vi "Decode Error.vi"(9 "cancel byte":u8, 10 "status byte":u8) -> (0 "Status":T1, 1 "Error message":string, 2 "Bad status byte?":bool, 3 "Error occured?":bool)   [LabVIEW 2023, in "Digikrom DK24x.lvlib"]
doc: "Decodes the status byte returned by the instrument."
uses:
  Digikrom DK24x.lvlib
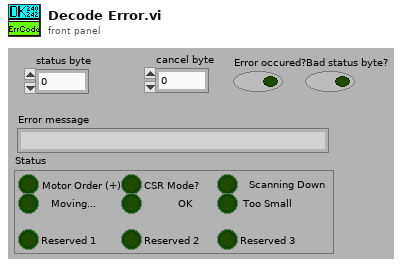
[diagram p1: front panel]
types:
  T1 = cluster{"Motor Order?":bool, "Reserved 1":bool, "CSR Mode?":bool, "Reserved 2":bool, "Scanning Up?":bool, "Too Large?":bool, "Already There?":bool, "Invalid Value?":bool, "Reserved 3":bool}
  T2 = cluster{"Boolean array[0]":bool, "Boolean array[1]":bool, "Boolean array[2]":bool, "Boolean array[3]":bool, "Boolean array[4]":bool, "Boolean array[5]":bool, "Boolean array[6]":bool, "Boolean array[7]":bool, "Boolean array[8]":bool}
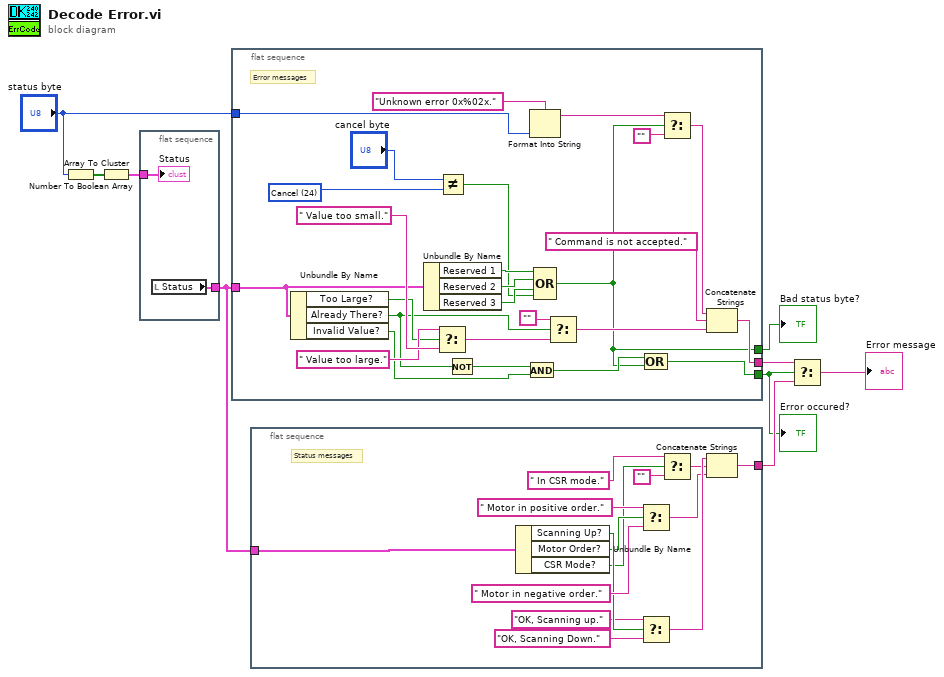
[diagram p0: block diagram]
diagram:
  n1 = Number To Boolean Array(number="status byte") -> (Boolean array=w7:bool[])
  n2 = Array To Cluster(array=w7) -> (cluster=w8:T2)
  n3 = flat-sequence {
    tunnel: [w10] -> w6
    tunnel: w8 -> [w11]
    frame #0 {
      n4 = local read "Status"() -> (w10:T1)
      "Status" <- w11
    }
  }
  n5 = flat-sequence {
    tunnel: [w37] -> w9
    tunnel: w6 -> [w23]
    tunnel: [w21] -> w4
    tunnel: [w17] -> w3
    tunnel: "status byte" -> [w15]
    frame #0 {
      w12 = u8 24 items=["Cancel"=24, "Clear"=25, "CSR"=28, "Echo"=27, "Filter"=15, "Gcal"=18, "Goto"=16, "Grtid?"=19, "Grtsel"=26, "NOVRAM Read"=56, "NOVRAM Write"=59, "Reset"=255, "Scan"=12, "Scan Up"=9, "Scan Down"=3, "Serial?"=33, "Slew Up"=8, "Slew Down"=2, "Slit Reset"=43, "Slit?"=30, "Sltadj"=14, "Speed"=13, "Sspeed?"=21, "Step Down"=1, "Step Up"=7, "S1adj"=31, "S2adj"=32, "S3adj"=34, "S1cal"=22, "S2cal"=23, "S3cal"=35, "Test"=17, "Type"=57, "Wave?"=29, "Zero"=52] ("Command")
      # "Error messages"
      n6 = Unbundle By Name(w23) -> ("Too Large?"=w28:bool, "Already There?"=w27:bool, "Invalid Value?"=w26:bool)
      n7 = Unbundle By Name(w23) -> ("Reserved 1"=w36:bool, "Reserved 2"=w35:bool, "Reserved 3"=w34:bool)
      n8 = Select(t=" Value too large.", s=w28, f=" Value too small.") -> (s? t:f=w32:string)
      n9 = Not Equal?(x="cancel byte", y=w12) -> (x != y?=w33:bool)
      n10 = Not(x=w27) -> (.not. x?=w25:bool)
      n11 = And(x=w25, y=w26) -> (x .and. y?=w22:bool)
      n12 = Format Into String(format string="Unknown error 0x%02x.", w15) -> (resulting string=w13:string)  [unwired: 2 in, 1 out]
      n13 = Compound Arithmetic op=OR(w36, w35, w34, w33) -> (w17:bool)
      n14 = Select(t="", s=w27, f=w32) -> (s? t:f=w19:string)
      n15 = Compound Arithmetic op=OR(w22, w17) -> (w21:bool)
      n16 = Select(t=w13, s=w17, f="") -> (s? t:f=w16:string)
      n17 = Concatenate Strings(w16, " Command is not accepted.", w19) -> (w37:string)
    }
  }
  n18 = flat-sequence {
    tunnel: w6 -> [w47]
    tunnel: [w40] -> w5
    frame #0 {
      # "Status messages"
      n19 = Unbundle By Name(w47) -> ("Scanning Up?"=w46:bool, "Motor Order?"=w45:bool, "CSR Mode?"=w44:bool)
      n20 = Select(t=" Motor in positive order.", s=w45, f=" Motor in negative order.") -> (s? t:f=w41:string)
      n21 = Select(t="OK, Scanning up.", s=w46, f="OK, Scanning Down.") -> (s? t:f=w43:string)
      n22 = Select(t=" In CSR mode.", s=w44, f="") -> (s? t:f=w42:string)
      n23 = Concatenate Strings(w43, w42, w41) -> (w40:string)
    }
  }
  n24 = Select(t=w9, s=w4, f=w5) -> (s? t:f=→"Error message":string)
  "Error occured?" <- w4
  "Bad status byte?" <- w3
